vi "Test Scaling.vi"() -> ()   [LabVIEW 2024]
uses:
  <vilib>/measure/NI_MABase.lvlib
panel:
  in  "Gain":dbl
  out "Waveform Graph":i16[][](graph)
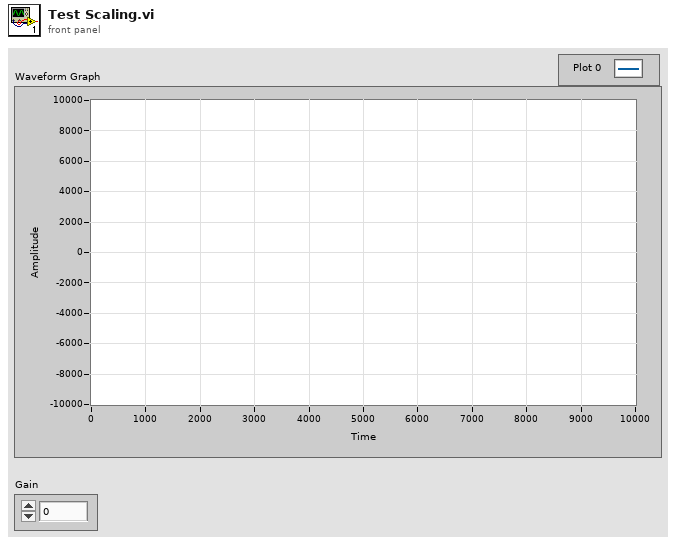
[diagram p1: front panel]
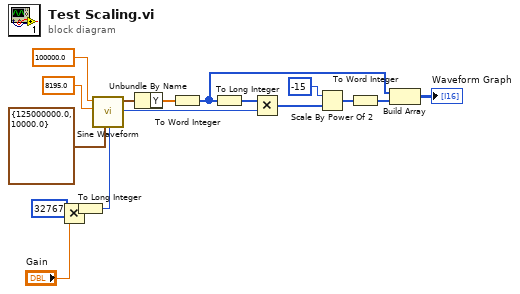
[diagram p0: block diagram]
diagram:
  n1 = Multiply(x=i16 32767, y="Gain") -> (x*y=w2:dbl)
  n2 = To Long Integer(number=w2) -> (32bit integer=w9:i32)
  n3 = call <vilib>:"Sine Waveform.vi"("sampling info"=cluster{"Fs":dbl, "#s":dbl} {"Fs"=125000000.0, "#s"=10000.0}, "amplitude"=8195.0, "frequency"=100000.0) -> ("signal out"=w13:waveform(dbl))  [unwired: 7 in, 1 out]
  n4 = Unbundle By Name(w13) -> ("Y"=w12:dbl[])
  n5 = To Word Integer(number=w12) -> (16bit integer=w7:i16[])
  n6 = To Long Integer(number=w7) -> (32bit integer=w10:i32[])
  n7 = Multiply(x=w10, y=w9) -> (x*y=w5:i32[])
  n8 = Scale By Power Of 2(n=i16 -15, x=w5) -> (x*2^n=w3:i32[])
  n9 = To Word Integer(number=w3) -> (16bit integer=w6:i16[])
  n10 = Build Array(w7, w6) -> (→"Waveform Graph":i16[][])
